vi "Read Device info parameters Ini file.vi"(8 "Error In":errorcluster, 11 "Read defaults":bool=TRUE) -> (0 "Error Out":errorcluster, 2 "Parameter names only":string[][](array[string]), 3 "Instrument info":string[][](array[string]), 4 "Cancelled":bool)   [LabVIEW 2020, in "Test Framework.lvclass"]
uses:
  Test Framework.lvclass
  <vilib>/Utility/config.llb/Read Key (String).vi
  <vilib>/Utility/config.llb/NI_LVConfig.lvlib
panel:
  out "Sizes of the sections":i32[](array[numeric])
  out "Sections read":string[](array[string])=["Instruments", "Environmental", "User"]
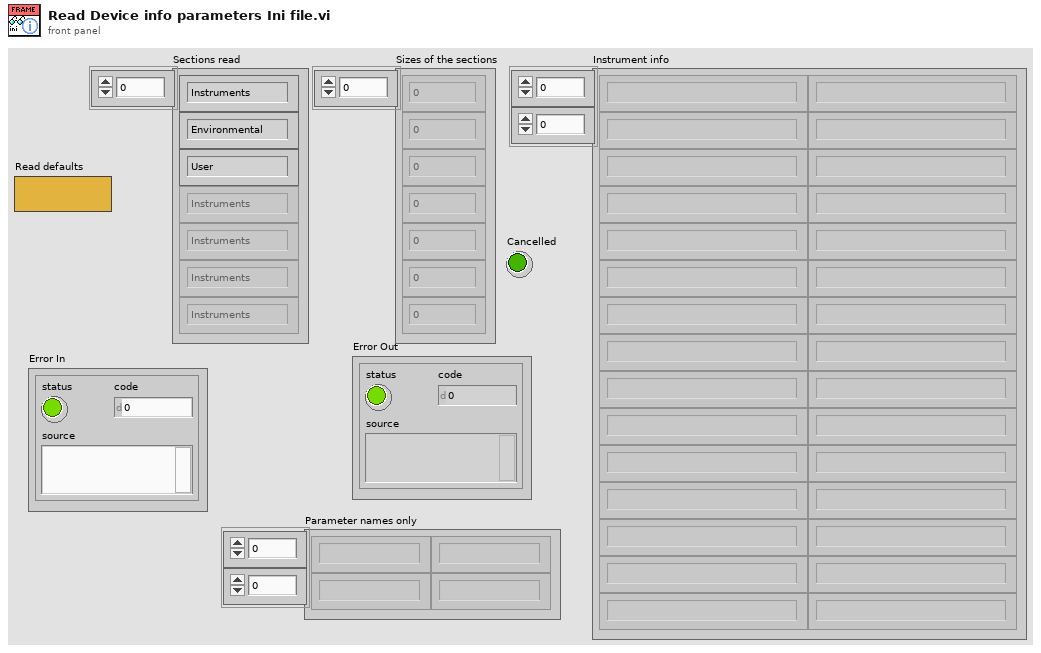
[diagram p1: front panel]
types:
  T1 = typedef "NI_LVConfig.lvlib/Config Data RefNum.ctl" = refnum<k1>
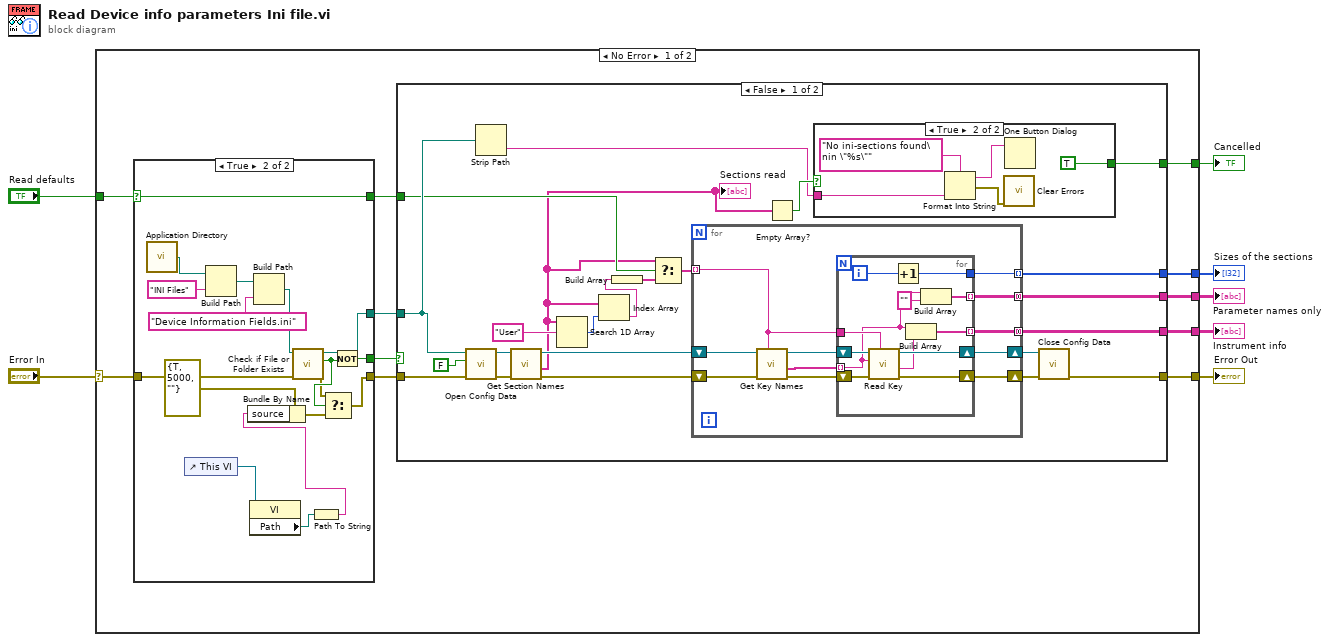
[diagram p0: block diagram]
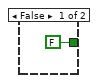
[diagram p2: hidden frame]
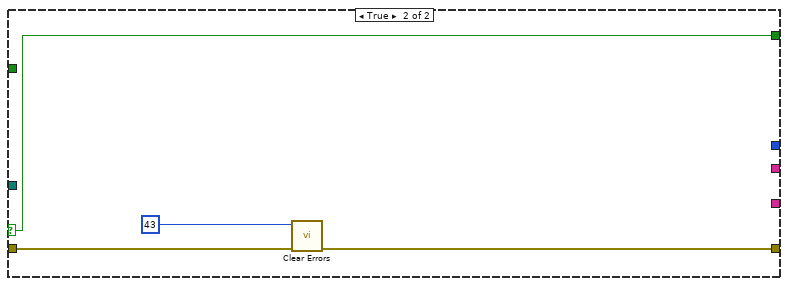
[diagram p3: hidden frame]
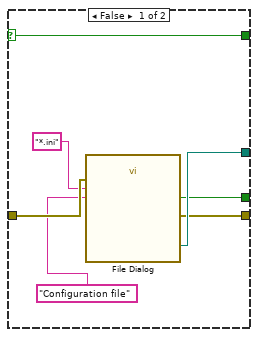
[diagram p4: hidden frame]
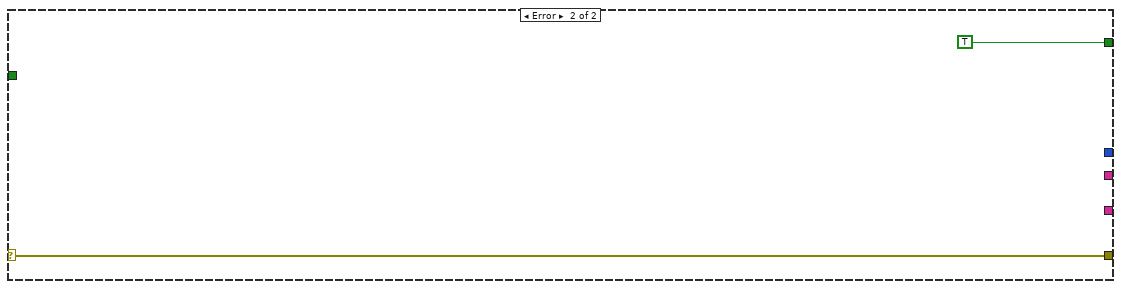
[diagram p5: hidden frame]
diagram:
  n1 = case shown="No Error" "Error In" {
    selector: "Error In" -> [w15 w100]
    tunnel: [w17 w100] -> w6
    tunnel: "Read defaults" -> [w16 _]
    tunnel: [w13 _] -> w4
    tunnel: [w12 _] -> w3
    tunnel: [w11 _] -> w2
    tunnel: [w9 TRUE] -> w1
    frame No Error {
      n2 = case shown="True" w16 {
        selector: w16 -> [w75 w82]
        tunnel: [w81 w93] -> w18
        tunnel: w15 -> [w80 w92]
        tunnel: [w79 w88] -> w14
        tunnel: [w78 w91] -> w10
        tunnel: [w75 w82] -> w8
        frame False {
          n3 = call "File Dialog"("error in"=w80, "pattern (all files)"="*.ini", "pattern label"="Configuration file") -> ("selected path"=w81:path, "cancelled"=w78:bool, "error out"=w79:errorcluster)  [unwired: 9 in, 1 out]
        }
        frame True {
          n4 = call <vilib>:"Application Directory.vi"() -> ("Application Directory"=w98:path)
          n5 = control-ref of="This VI"() -> (w85:refnum<vi>)
          n6 = Build Path(base path=w98, name or relative path="INI Files") -> (appended path=w96:path)
          n7 = property class="VI"(reference=w85) -> ("Path"=w84:path)  [unwired: 1 in, 2 out]
          n8 = Build Path(base path=w96, name or relative path="Device Information Fields.ini") -> (appended path=w94:path)
          n9 = call <vilib>:"Check if File or Folder Exists.vi"("error in (no error)"=w92, "path"=w94) -> ("error out"=w89:errorcluster, "file or folder exists?"=w90:bool, "dup path"=w93:path)  [unwired: 7 in]
          n10 = Path To String(path=w84) -> (string=w83:string)
          n11 = Bundle By Name(cluster=errorcluster {"status"=TRUE, "code"=5000, "source"=""} ("error constant"), "source"=w83) -> (w86:errorcluster)
          n12 = Select(t=w89, s=w90, f=w86) -> (s? t:f=w88:errorcluster)
          n13 = Not(x=w90) -> (.not. x?=w91:bool)
        }
      }
      n14 = case shown="False" w10 {
        selector: w10 -> [_ w71]
        tunnel: w18 -> [w28 _]
        tunnel: [w40 w73] -> w17
        tunnel: w14 -> [w33 w74]
        tunnel: [w32 _] -> w13
        tunnel: [w31 _] -> w12
        tunnel: [w30 _] -> w11
        tunnel: [w26 w71] -> w9
        tunnel: w8 -> [w23 _]
        frame False {
          n15 = call <vilib>:"Open Config Data.vi"("error in (no error)"=w33, "create file if necessary (T)"=FALSE, "configuration file path"=w28) -> ("error out"=w38:errorcluster, "refnum"=w37:T1)  [unwired: 6 in, 1 out]
          n16 = Strip Path(path=w28) -> (name=w27:string)  [unwired: 1 out]
          n17 = call <vilib>:"Get Section Names.vi"("error in (no error)"=w38, "refnum"=w37) -> ("error out"=w35:errorcluster, "section names"=w22:string[], "refnum out"=w36:T1)  [unwired: 7 in]
          "Sections read" <- w22
          n18 = Search 1D Array(1D array=w22, element="User") -> (index of element=w24:i32)  [unwired: 1 in]
          n19 = Index Array(array=w22, index=w24) -> (element=w19:string)
          n20 = Build Array(w19) -> (w20:string[])
          n21 = Select(t=w22, s=w23, f=w20) -> (s? t:f=w21:string[])
          n22 = for {
            tunnel: w21 -> [w53] mode=indexing
            shift-right: [w52] -> w41
            shift-left: w35 -> [w58]
            tunnel: [w51] -> w30 mode=indexing
            shift-right: [w50] -> w39
            shift-left: w36 -> [w57]
            tunnel: [w49] -> w32 mode=concatenating
            tunnel: [w48] -> w31 mode=concatenating
            n23 = call <vilib>:"Get Key Names.vi"("section"=w53, "error in (no error)"=w58, "refnum"=w57) -> ("error out"=w56:errorcluster, "key names"=w55:string[], "refnum out"=w54:T1)  [unwired: 5 in, 1 out]
            n24 = for {
              shift-right: [w69] -> w52
              shift-left: w56 -> [w70]
              tunnel: w55 -> [w61] mode=indexing
              tunnel: w53 -> [w64]
              tunnel: [w63] -> w48 mode=indexing
              tunnel: [w65] -> w51
              shift-right: [w67] -> w50
              shift-left: w54 -> [w68]
              tunnel: [w60] -> w49 mode=indexing
              i -> [w66]
              n25 = call-poly <vilib>:"Read Key.vi"("section"=w64, "error in (no error)"=w70, "key"=w61, "refnum"=w68) -> ("error out"=w69:errorcluster, "value"=w62:string, "refnum out"=w67:T1)  [unwired: 4 in, 1 out]
              n26 = Increment(x=w66) -> (x+1=w65:i32)
              n27 = Build Array(w61, w62) -> (w63:string[])
              n28 = Build Array(w61, "" ("element")) -> (w60:string[])
            }
          }
          n29 = Empty Array?(array=w22) -> (empty?=w29:bool)
          n30 = case shown="True" w29 {
            tunnel: w27 -> [_ w44]
            tunnel: [FALSE TRUE] -> w26
            frame False {
            }
            frame True {
              n31 = Format Into String(format string="No ini-sections found\nin \"%s\"" ("message"), w44) -> (resulting string=w46:string, error out=w45:errorcluster)  [unwired: 2 in]
              n32 = call <vilib>:"Clear Errors.vi"("error in (no error)"=w45) -> ()  [unwired: 5 in, 2 out]
              n33 = One Button Dialog(message=w46) -> ()  [unwired: 1 in, 1 out]
            }
          }
          n34 = call <vilib>:"Close Config Data.vi"("error in (no error)"=w41, "refnum"=w39) -> ("error out"=w40:errorcluster)  [unwired: 8 in, 1 out]
        }
        frame True {
          n35 = call <vilib>:"Clear Errors.vi"("error in (no error)"=w74, "specific error code to clear (0: all)"=43) -> ("error out"=w73:errorcluster)  [unwired: 4 in, 1 out]
        }
      }
    }
    frame Error {
    }
  }
  "Error Out" <- w6
  "Sizes of the sections" <- w2
  "Instrument info" <- w3
  "Parameter names only" <- w4
  "Cancelled" <- w1
